vi "Interpolate Climb System.vi"(8 "Duration":dbl, 9 "Current Time":dbl, 10 "End Climb Motor Commands":T1, 11 "Start Climb Motor Commands":T1) -> (3 "Current Climb Motor Commands":T1)   [LabVIEW 2018]
uses:
  Controls/Climb Motor Commands.ctl
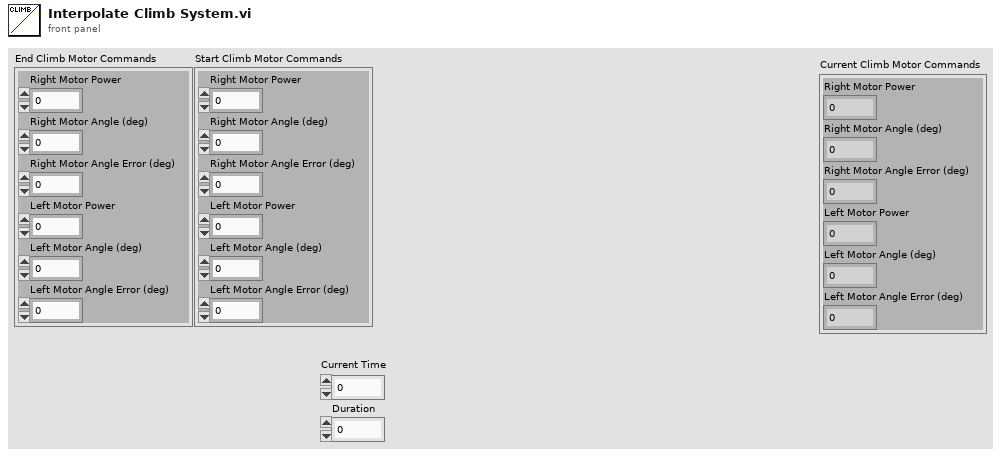
[diagram p1: front panel]
types:
  T1 = typedef "Climb Motor Commands.ctl" = cluster{"Right Motor Power":dbl, "Right Motor Angle (deg)":dbl, "Right Motor Angle Error (deg)":dbl, "Left Motor Power":dbl, "Left Motor Angle (deg)":dbl, "Left Motor Angle Error (deg)":dbl}
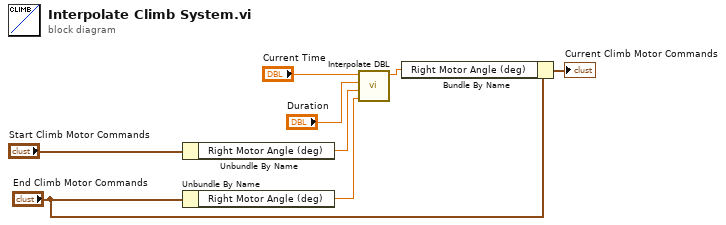
[diagram p0: block diagram]
diagram:
  n1 = Unbundle By Name("Start Climb Motor Commands") -> ("Right Motor Angle (deg)"=w3:dbl)
  n2 = Unbundle By Name("End Climb Motor Commands") -> ("Right Motor Angle (deg)"=w2:dbl)
  n3 = call "Interpolate DBL.vi"("Ending Value"=w2, "Starting Value"=w3, "Duration"="Duration", "Current Time"="Current Time") -> ("Current Value"=w1:dbl)  [unwired: 7 in]
  n4 = Bundle By Name(cluster="End Climb Motor Commands", "Right Motor Angle (deg)"=w1) -> (→"Current Climb Motor Commands":T1)
